vi "Global - Server.vi"() -> ()   [LabVIEW 2024]
doc: "Stores the global data for the server."
uses:
  Controls/Server/Subsystem IO Attributes.ctl
  Controls/Server/Subsystem IO Logging Attributes.ctl
  Controls/Server/Subsystem IO Alarm Attributes.ctl
  Controls/Server/System Configuration.ctl
  Controls/Server/Subsystem Configuration.ctl
panel:
  in  "System Configuration":refnum<data-value>
  in  "Subsystem I/O Attributes":refnum<data-value> caption="Subsystem Attributes Value Reference"
  in  "Subsystem I/O Attributes File":path
  in  "System Configuration File":path
  # "The Global - Server.vi stores the global data for the server. The global data includes the static configurations and data that are not changed frequently and can be visited from anywhere in the code."
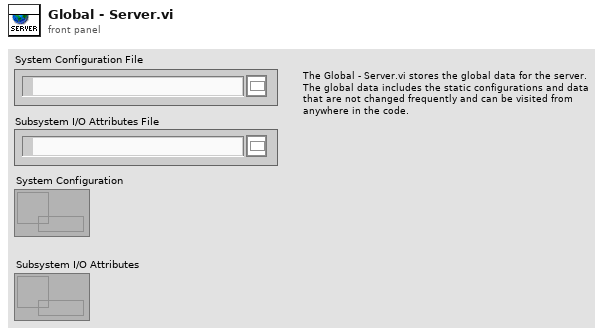
[diagram p1: front panel]
diagram:
